vi "Autonomous.vi"   [LabVIEW 2017]
doc: "This VI starts when autonomous period begins, and will automatically be terminated when it ends. You can carry out timed or sensor driven operations directly to I/O or to subsystems without needing to return to the caller."
uses:
  <vilib>/Rock Robotics/Network Tables/NT Read Numeric Array.vi
  <vilib>/Rock Robotics/Network Tables/NT Read Number.vi
  <vilib>/Rock Robotics/Network Tables/NT Read Boolean.vi
  <vilib>/Rock Robotics/Network Tables/NT Write String.vi
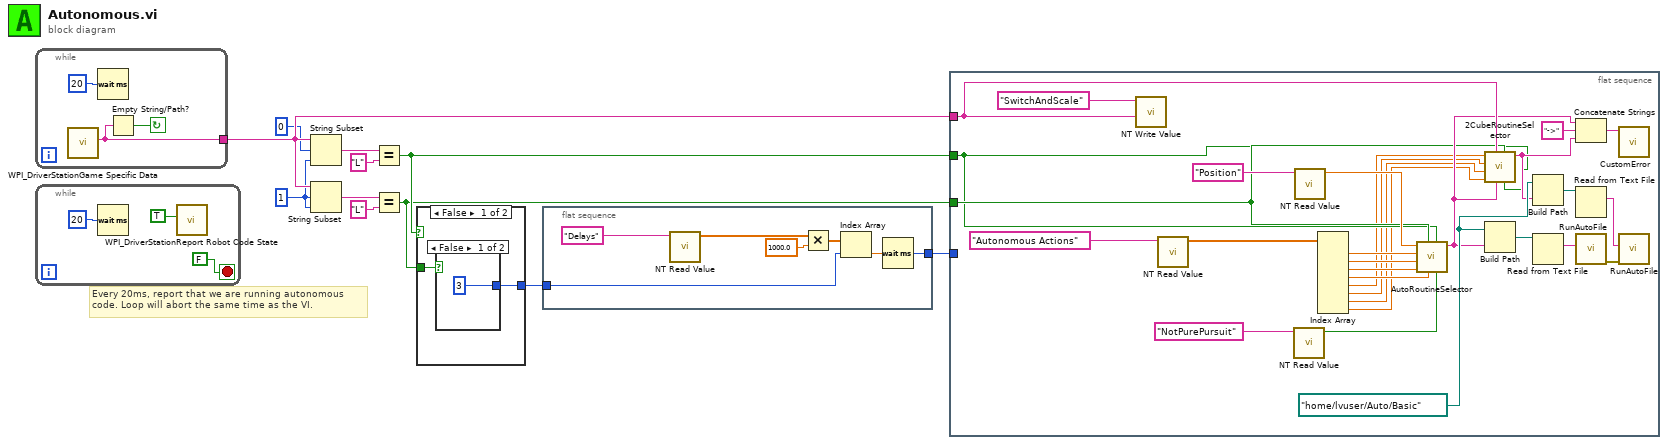
[diagram p0: block diagram]
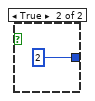
[diagram p2: hidden frame]
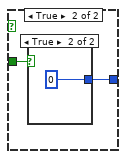
[diagram p3: hidden frame]
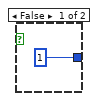
[diagram p4: hidden frame]
diagram:
  w6 = 1 ("length (rest)")
  # "Every 20ms, report that we are running autonomous\ncode. Loop will abort the same time as the VI."
  n1 = while {
    tunnel: [w14] -> w11
    stop <- w13 continue-if-true
    n2 = call <vilib>:"WPI_DriverStationGame Specific Data.vi"() -> ("Game Specific Data"=w14:string)  [unwired: 11 in]
    n3 = Wait (ms)(milliseconds to wait=u32 20) -> ()  [unwired: 1 out]
    n4 = Empty String/Path?(string/path=w14) -> (empty?=w13:bool)
  }
  n5 = while {
    stop <- FALSE stop-if-true
    n6 = Wait (ms)(milliseconds to wait=u32 20) -> ()  [unwired: 1 out]
    n7 = call <vilib>:"WPI_DriverStationReport Robot Code State.vi"("Autonomous"=TRUE) -> ()  [unwired: 10 in, 1 out]
  }
  n8 = String Subset(string=w11, offset (0)=0 ("length (rest)"), length (rest)=w6) -> (substring=w9:string)
  n9 = String Subset(string=w11, offset (0)=w6, length (rest)=w6) -> (substring=w10:string)
  n10 = Equal?(x=w9, y="L") -> (x = y?=w4:bool)
  n11 = Equal?(x=w10, y="L") -> (x = y?=w3:bool)
  n12 = case shown="False" w4 {
    tunnel: w3 -> [w19 w23]
    tunnel: [w18 w22] -> w1
    frame False {
      n13 = case shown="False" w19 {
        tunnel: [3 2] -> w18
        frame False {
        }
        frame True {
        }
      }
    }
    frame True {
      n14 = case shown="True" w23 {
        tunnel: [1 0] -> w22
        frame False {
        }
        frame True {
        }
      }
    }
  }
  n15 = flat-sequence {
    tunnel: w1 -> [w27]
    tunnel: [w26] -> w2
    frame #0 {
      n16 = call-poly <vilib>:"NT Read Value.vi"("Name"="Delays") -> ("Numeric Array"=w32:dbl[])  [unwired: 9 in, 1 out]
      n17 = Multiply(x=w32, y=1000.0) -> (x*y=w29:dbl[])
      n18 = Index Array(array=w29, index=w27) -> (element=w28:dbl)
      n19 = Wait (ms)(milliseconds to wait=w28) -> (millisecond timer value=w26:u32)
    }
  }
  n20 = flat-sequence {
    tunnel: w11 -> [w55]
    tunnel: w3 -> [w38]
    tunnel: w4 -> [w37]
    tunnel: w2 -> [_]
    frame #0 {
      w52 = path "/home/lvuser/Auto/Basic" ("base path")
      n21 = call-poly <vilib>:"NT Write Value.vi"("String"=w55, "Name"="SwitchAndScale") -> ()  [unwired: 9 in, 1 out]
      n22 = call-poly <vilib>:"NT Read Value.vi"("Name"="Autonomous Actions") -> ("Numeric Array"=w45:dbl[])  [unwired: 9 in, 1 out]
      n23 = call-poly <vilib>:"NT Read Value.vi"("Name"="NotPurePursuit") -> ("Boolean"=w44:bool)  [unwired: 9 in, 1 out]
      n24 = call-poly <vilib>:"NT Read Value.vi"("Name"="Position") -> ("Numeric"=w50:dbl)  [unwired: 9 in, 1 out]
      n25 = Index Array(array=w45) -> (element #1=w43:dbl, element #2=w42:dbl, element #3=w41:dbl, element #4=w40:dbl, element #5=w36:dbl, element #6=w35:dbl, element #7=w34:dbl, element #8=w33:dbl)  [unwired: 8 in]
      n26 = call "AutoRoutineSelector.vi"("NotPurePursuit"=w44, "OurSwitch"=w37, "RR"=w40, "OurScale"=w38, "RL"=w41, "LR"=w42, "LL"=w43, "Position"=w50) -> ("File Name"=w39:string)  [unwired: 3 in]
      n27 = call "2CubeRoutineSelector.vi"("Switch"=w37, "Scale"=w38, "Prior Routine File Name"=w39, "GameData"=w55, "RR"=w33, "RL"=w34, "LR"=w35, "LL"=w36) -> ("File Path"=w48:string)  [unwired: 3 in]
      n28 = Build Path(base path=w52, name or relative path=w39) -> (appended path=w58:path)
      n29 = Build Path(base path=w52, name or relative path=w48) -> (appended path=w53:path)
      n30 = Read from Text File(file (use dialog)=w58) -> (text=w57:string)  [unwired: 3 in, 3 out]
      n31 = Concatenate Strings(w39, "->" ("string"), w48) -> (w47:string)
      n32 = Read from Text File(file (use dialog)=w53) -> (text=w54:string)  [unwired: 3 in, 3 out]
      n33 = call "RunAutoFile.vi"("AutoFile"=w57) -> ("error out"=w51:errorcluster)  [unwired: 10 in]
      n34 = call "CustomError.vi"("String"=w47) -> ()  [unwired: 10 in, 1 out]
      n35 = call "RunAutoFile.vi"("error in (no error)"=w51, "AutoFile"=w54) -> ()  [unwired: 9 in, 1 out]
    }
  }
